vi "UnOrFormat Alarm.vi"(8 "error in (no error)":errorcluster, 9 "Alarm String Array In":string[][](array[string]), 10 "Direction":T2, 11 "Alarms List In":T1[](array[typedef])) -> (0 "error out":errorcluster, 1 "Alarms List Out":T1[](array[typedef]), 3 "Alarm String Array Out":string[][](array[string]))   [LabVIEW 2017]
uses:
  AlarmElementControl.ctl
  AlarmConvertDirectionEnumControl.ctl
  myDateTimeRecCluster.ctl
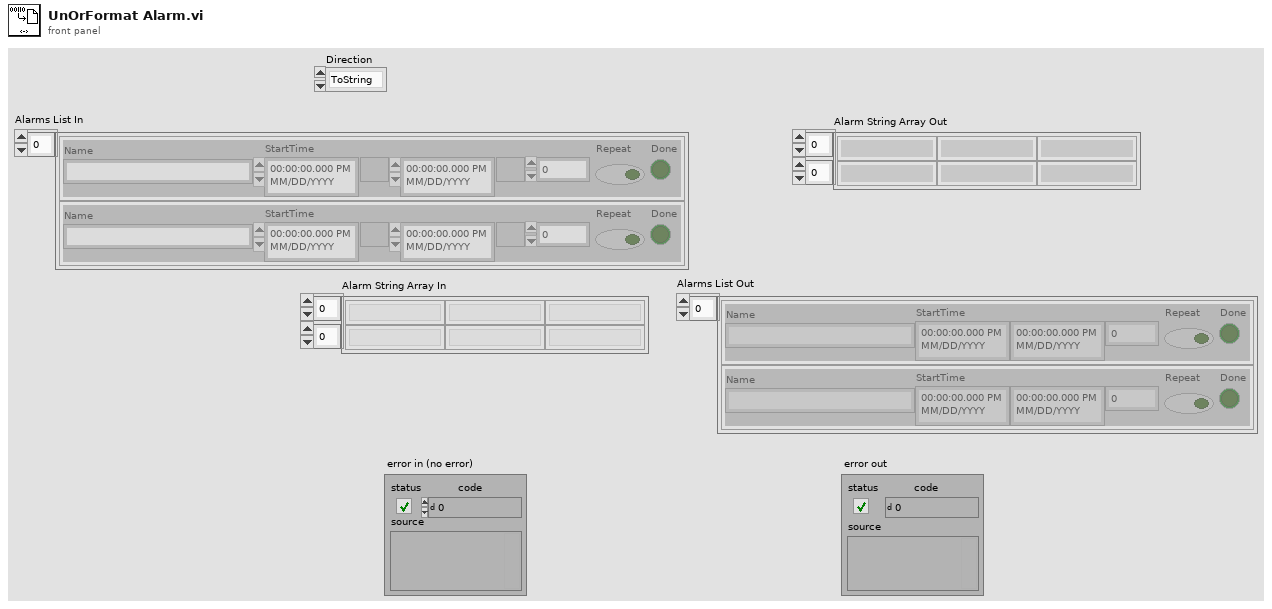
[diagram p1: front panel]
types:
  T1 = typedef "AlarmElementControl.ctl" = cluster{"Name":string, "StartTime ":timestamp, "End Time":timestamp, "Duration":i32, "Repeat":bool, "Done":bool}
  T2 = typedef "AlarmConvertDirectionEnumControl.ctl" = enum16{"ToString", "ToCluster"}
  T3 = typedef "LVDateTimeRec.ctl" = cluster{"fractional second":dbl, "second":i32, "minute":i32, "hour":i32, "day of month":i32, "month":i32, "year":i32, "day of week":i32, "day of year":i32, "DST":i32}
  T4 = typedef "myDateTimeRecCluster.ctl" = cluster{"Frac Sec":dbl, "Sec":i32, "Min":i32, "Hr":i32, "DoMth":i32, "Mth":i32, "Yr":i32, "DoWk":i32, "DoYr":i32, "DST":i32}
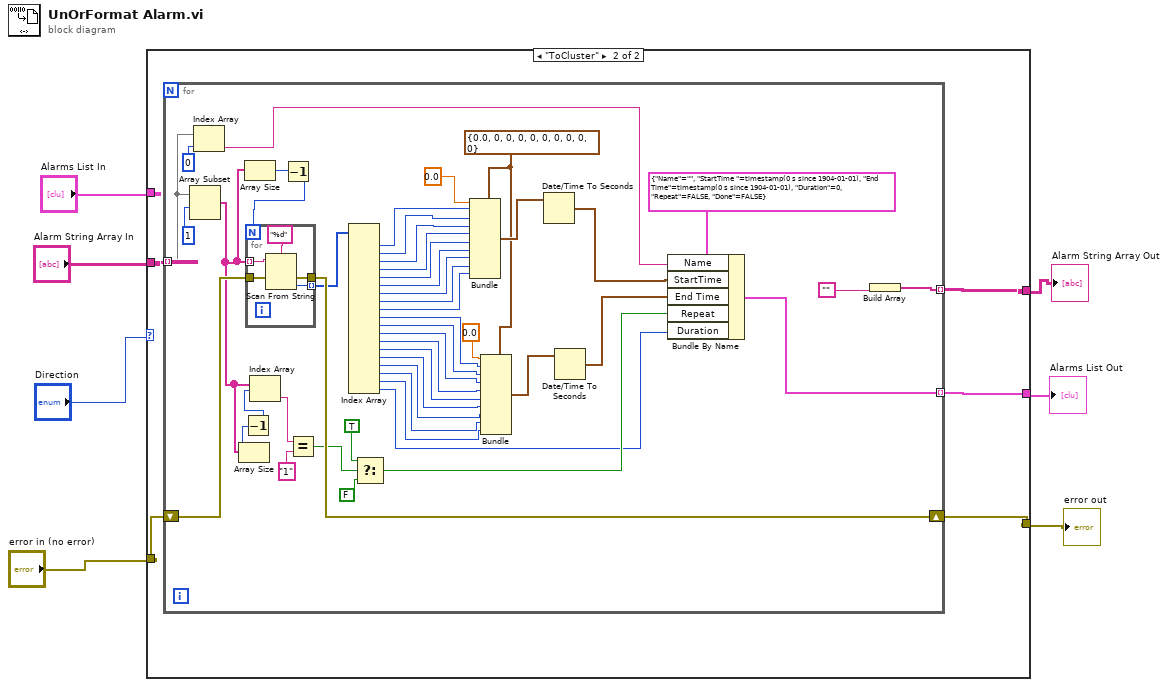
[diagram p0: block diagram]
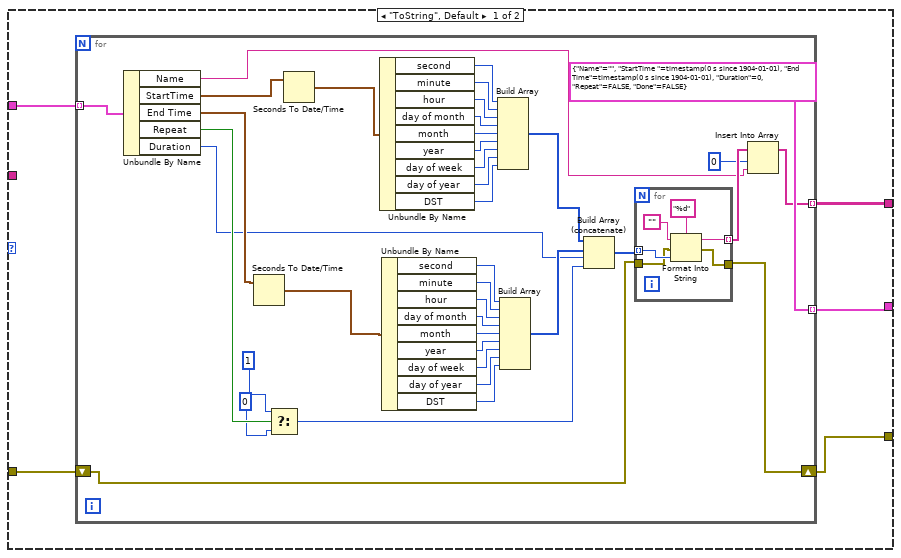
[diagram p2: hidden frame]
diagram:
  n1 = case shown="\"ToCluster\"" "Direction" {
    tunnel: "Alarms List In" -> [w9 _]
    tunnel: "error in (no error)" -> [w8 w60]
    tunnel: [w12 w61] -> w1
    tunnel: [w11 w59] -> w2
    tunnel: "Alarm String Array In" -> [_ w58]
    tunnel: [w10 w57] -> w3
    frame "ToString", Default {
      n2 = for {
        tunnel: [w15] -> w12 mode=indexing
        tunnel: [T1 {"Name"="", "StartTime "=timestamp(0 s since 1904-01-01), "End Time"=timestamp(0 s since 1904-01-01), "Duration"=0, "Repeat"=FALSE, "Done"=FALSE} ("Alarm")] -> w10 mode=indexing
        tunnel: w9 -> [w19] mode=indexing
        shift-right: [w21] -> w11
        shift-left: w8 -> [w22]
        n3 = Unbundle By Name(w19) -> ("Name"=w16:string, "StartTime"=w50:timestamp, "End Time"=w49:timestamp, "Repeat"=w26:bool, "Duration"=w13:i32)
        n4 = Seconds To Date/Time(time stamp (now)=w49) -> (date time rec=w29:T3)  [unwired: 1 in]
        n5 = Select(t=1, s=w26, f=0) -> (s? t:f=w14:i32)
        n6 = Seconds To Date/Time(time stamp (now)=w50) -> (date time rec=w48:T3)  [unwired: 1 in]
        n7 = Unbundle By Name(w48) -> ("second"=w47:i32, "minute"=w46:i32, "hour"=w45:i32, "day of month"=w44:i32, "month"=w43:i32, "year"=w42:i32, "day of week"=w41:i32, "day of year"=w40:i32, "DST"=w39:i32)
        n8 = Unbundle By Name(w29) -> ("second"=w38:i32, "minute"=w37:i32, "hour"=w36:i32, "day of month"=w35:i32, "month"=w34:i32, "year"=w33:i32, "day of week"=w32:i32, "day of year"=w31:i32, "DST"=w30:i32)
        n9 = Build Array(w47, w46, w45, w44, w43, w42, w41, w40, w39) -> (w28:i32[])
        n10 = Build Array(w38, w37, w36, w35, w34, w33, w32, w31, w30) -> (w27:i32[])
        n11 = Build Array (concatenate)(w28, w27, w13, w14) -> (w23:i32[])
        n12 = for {
          tunnel: w23 -> [w56] mode=indexing
          tunnel: w22 -> [w55]
          tunnel: [w52] -> w21
          tunnel: [w51] -> w18 mode=indexing
          n13 = Format Into String(format string="%d", initial string="", error in=w55, w56) -> (resulting string=w51:string, error out=w52:errorcluster)
        }
        n14 = Insert Into Array(array=w18, index=0, new element=w16) -> (w15:string[])
      }
    }
    frame "ToCluster" {
      n15 = for {
        tunnel: [w108] -> w61 mode=indexing
        tunnel: w58 -> [w65] mode=indexing
        tunnel: [w72] -> w57 mode=indexing
        shift-right: [w106] -> w59
        shift-left: w60 -> [w107]
        w92 = T4 {"Frac Sec"=0.0, "Sec"=0, "Min"=0, "Hr"=0, "DoMth"=0, "Mth"=0, "Yr"=0, "DoWk"=0, "DoYr"=0, "DST"=0}
        n16 = Array Subset(array=w65, index=1) -> (w66:string[])  [unwired: 1 in]
        n17 = Index Array(array=w65, index=0) -> (element=w63:string)
        n18 = Array Size(array=w66) -> (size(s)=w71:i32)
        n19 = Decrement(x=w71) -> (x-1=w70:i32)
        n20 = Array Size(array=w66) -> (size(s)=w69:i32)
        n21 = Index Array(array=w66, index=w70) -> (element=w81:string)
        n22 = Decrement(x=w69) -> (x-1=w68:i32)
        n23 = for {
          N: w68 -> [_]
          tunnel: w66 -> [w114] mode=indexing
          tunnel: w107 -> [w112]
          tunnel: [w111] -> w106
          tunnel: [w110] -> w105 mode=indexing
          n24 = Scan From String(format string="%d", input string=w114, error in=w112) -> (error out=w111:errorcluster, output 1=w110:i32)  [unwired: 2 in, 2 out]
        }
        n25 = Equal?(x=w81, y="1") -> (x = y?=w79:bool)
        n26 = Index Array(array=w105) -> (element #1=w104:i32, element #2=w103:i32, element #3=w102:i32, element #4=w101:i32, element #5=w100:i32, element #6=w99:i32, element #7=w98:i32, element #8=w97:i32, element #9=w96:i32, element #10=w90:i32, element #11=w89:i32, element #12=w88:i32, element #13=w87:i32, element #14=w86:i32, element #15=w85:i32, element #16=w84:i32, element #17=w83:i32, element #18=w82:i32, element #19=w62:i32)  [unwired: 19 in]
        n27 = Select(t=TRUE, s=w79, f=FALSE) -> (s? t:f=w73:bool)
        n28 = Bundle(cluster=w92, "Frac Sec"=0.0, "Sec"=w104, "Min"=w103, "Hr"=w102, "DoMth"=w101, "Mth"=w100, "Yr"=w99, "DoWk"=w98, "DoYr"=w97, "DST"=w96) -> (w94:T4)
        n29 = Bundle(cluster=w92, "Frac Sec"=0.0, "Sec"=w90, "Min"=w89, "Hr"=w88, "DoMth"=w87, "Mth"=w86, "Yr"=w85, "DoWk"=w84, "DoYr"=w83, "DST"=w82) -> (w93:T4)
        n30 = Date/Time To Seconds(2:w94) -> (0:w75:timestamp)  [unwired: 1 in]
        n31 = Date/Time To Seconds(2:w93) -> (0:w74:timestamp)  [unwired: 1 in]
        n32 = Bundle By Name(cluster=T1 {"Name"="", "StartTime "=timestamp(0 s since 1904-01-01), "End Time"=timestamp(0 s since 1904-01-01), "Duration"=0, "Repeat"=FALSE, "Done"=FALSE} ("Alarm"), "Name"=w63, "StartTime"=w75, "End Time"=w74, "Repeat"=w73, "Duration"=w62) -> (w72:T1)
        n33 = Build Array("") -> (w108:string[])
      }
    }
  }
  "Alarm String Array Out" <- w1
  "error out" <- w2
  "Alarms List Out" <- w3
